vi "Simulation - Lead-Lag.vi"() -> ()   [LabVIEW 2023]
doc: "This VI demonstrates the PID Lead-Lag VI. You can tune the parameters and watch the behavior on the Process Signals graph."
uses:
  <vilib>/addons/control/pid/pid.llb/PID Lead-Lag (DBL).vi
  <vilib>/addons/control/pid/NI_PID_pid.lvlib
panel:
  in  "Tab Control":enum32{"Lead or Lag", "Raw Parameters"}(tab)
  in  "Type of Parameters":u16(ring)=1 items=["Lead", "Lag"]
  in  "Gain":dbl(slide)=0.75 scale=0.01..10.0
  in  "Time constant":dbl(knob)=0.002 scale=0.0001..1.0
  in  "Tuning Parameters":T1={"Gain"=1.0, "Lag time (min)"=0.01, "Lead time (min)"=0.001} {"Lead time (min)" format="%.3f"; "Lag time (min)" format="%.3f"; "Gain" format="%.3f"}
  in  "output range":cluster{"output high":dbl, "output low":dbl}={"output high"=400.0, "output low"=-400.0} {"output low" format="%.2f"; "output high" format="%.2f"}
  in  "Lead-Lag Unit Time":u16(ring)=1 items=["second", "minute"]
  in  "Stop":bool
  out "Process Signals":cluster{dbl, "output":dbl}(graph)={48.67085016096563, "output"=100.0}
  in  "Input Signal":u16(ring) items=["Sine", "Square"]
  # "Overview: This VI demonstrates the PID Lead-Lag VI.  You can tune the parameters and watch the behavior on the Process Signals graph.\nInstructions:\n1. Run the VI and verify the input waveform and the output signal on the Lead-Lag function.\n2. Choose the Input signal as Sine and verify that the output of the lead-lag have the phase of the sine wave leading (ahead) or lagging (behind) the input signal.\n3. Change the Input signal to Square and change the Parameters to tab to Raw parameters. This will show the combination of lead and lag parameters.\n4. Change the output range and verify how that affects the limits of the output signal.\n5. Click Stop to stop the VI."
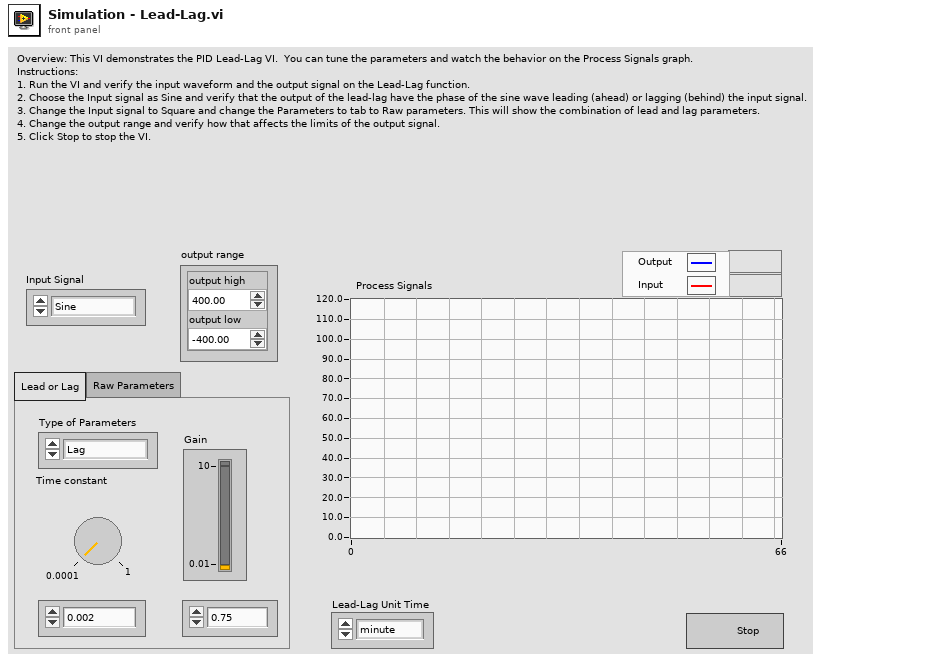
[diagram p1: front panel]
types:
  T1 = cluster{"Gain":dbl, "Lag time (min)":dbl, "Lead time (min)":dbl}
  T2 = cluster{"Gain":dbl, "Time constant":dbl, "Time constant":dbl}
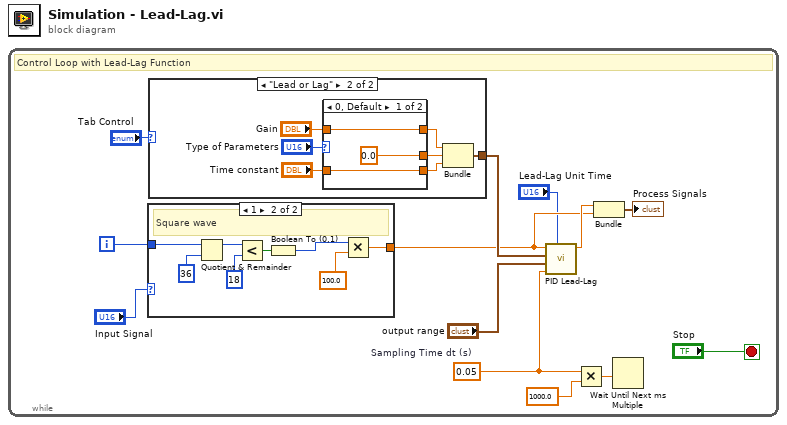
[diagram p0: block diagram]
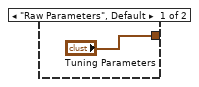
[diagram p2: hidden frame]
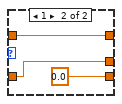
[diagram p3: hidden frame]
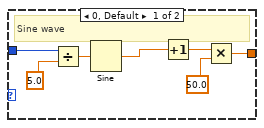
[diagram p4: hidden frame]
diagram:
  n1 = while {
    i -> [w9]
    stop <- "Stop" stop-if-true
    w2 = 0.05  # Sampling Time dt (s)
    # "Control Loop with Lead-Lag Function"
    n2 = case shown="1" "Input Signal" {
      tunnel: [w30 w39] -> w7
      tunnel: w9 -> [w29 w42]
      frame 0, Default {
        # "Sine wave"
        n3 = Divide(x=w29, y=5.0) -> (x/y=w32:dbl)
        n4 = Sine(x=w32) -> (sin(x)=w28:dbl)
        n5 = Increment(x=w28) -> (x+1=w33:dbl)
        n6 = Multiply(x=w33, y=50.0) -> (x*y=w30:dbl)
      }
      frame 1 {
        # "Square wave"
        n7 = Quotient & Remainder(x=w42, y=36) -> (x-y*floor(x/y)=w38:i32)  [unwired: 1 out]
        n8 = Less?(x=w38, y=18) -> (x < y?=w36:bool)
        n9 = Boolean To (0,1)(Boolean=w36) -> (0, 1=w35:i16)
        n10 = Multiply(x=w35, y=100.0) -> (x*y=w39:dbl)
      }
    }
    n11 = case shown="\"Lead or Lag\"" "Tab Control" {
      tunnel: ["Tuning Parameters" w17] -> w10
      frame "Raw Parameters", Default {
      }
      frame "Lead or Lag" {
        n12 = case shown="0, Default" "Type of Parameters" {
          tunnel: [0.0 ("Time constant") w26] -> w20
          tunnel: "Time constant" -> [w23 w26]
          tunnel: [w23 0.0] -> w18
          tunnel: [w22 w25] -> w16
          tunnel: "Gain" -> [w22 w25]
          frame 0, Default {
          }
          frame 1 {
          }
        }
        n13 = Bundle("Gain"=w16, "Time constant"=w20, "Time constant"=w18) -> (w17:T2)  [unwired: 1 in]
      }
    }
    n14 = call-poly <vilib>:"PID Lead-Lag.vi"("time unit"="Lead-Lag Unit Time", "dt (s)"=w2, "output range"="output range", "tuning parameters"=w10, "input"=w7) -> ("output"=w8:dbl)  [unwired: 3 in, 1 out]
    n15 = Multiply(x=w2, y=1000.0) -> (x*y=w11:dbl)
    n16 = Bundle("output"=w8, w7) -> (→"Process Signals":cluster{"output":dbl, dbl})  [unwired: 1 in]
    n17 = Wait Until Next ms Multiple(millisecond multiple=w11) -> ()  [unwired: 1 out]
  }
